vi "camera_grayscale.vi"(0 "Camera configuration":string="{\n     \"type\": \"Camera\",\n     \"listen_port\": 8012,\n     \"location\": {\n       \"x\": 0.0,\n       \"y\": 0.0,\n       \"z\": 250.0\n     },\n     \"rotation\": {\n       \"pitch\": 0.0,\n       \"yaw\": 0.0,\n       \"roll\": 0.0\n     },\n     \"stream_dimensions\": {\n       \"x\": 512.0,\n       \"y\": 512.0\n     },\n    \"dynamic_range\": 1.0,\n   \t\"fov\": 60.0,\n    \"camera_matrix\": [\n         [433.0, 0.0,   256.0],\n         [0.0,   433.0, 256.0],\n         [0.0,   0.0,   1.0]\n     ],\t\n   \t\"min_shutter\": 0.0005,\n   \t\"max_shutter\": 0.0014,\n    \"motion_blur_bias\": 0.1,\n    \"white_balance\": 0.0,\n    \"white_balance_temp_offset\": 0,\n    \"exposure_compensation\": -1.0,\n    \"image_noise_bias\": 0.05,\n    \"ray_tracing\":{\n       \"enable_ray_tracing\": false\n    },\n   \"channels\" : \"gray\",\n   \"annotation\": {\n      \"include_annotation\": false,\n      \"desired_tags\": [\n        \"traffic_sign\", \"vehicle\"\n      ],\n     \"include_lanes\": true,\n\t\t    \"lane_sampling_distance\": 15000.0,\n\t\t    \"lane_sampling_frequency\": 100.0,\n\t\t    \"lane_subsampling\": 10.0,\n      \"far_plane\": 10000.0,\n      \"include_tags\": true,\n      \"include_obb\": false,\n      \"cull_partial_frame\":false,\n      \"debug_draw\":false\n    },\n    \"max_distance\":50000.0,\n    \"channel_depth\":1\n}\n", 3 "error In":errorcluster={"status"=FALSE, "code"=0, "source"="Event Code: 0\r\n\r\n-----------------------------------\nEvent Code: 0\r\n{\"message\":\"Successfully configured scenario.\",\"reference\":973,\"success\":true,\"type\":\"ClosedLoopConfigCommand_ID\"}\r\n-----------------------------------\nEvent Code: 0\r\n{\"message\":\"weather configured to \\\"Default\\\"\",\"reference\":703,\"success\":true,\"type\":\"WeatherConfig\"}\r\n-----------------------------------\nEvent Code: 0\r\n{\"message\":\"complete\",\"reference\":874,\"success\":true,\"type\":\"REPLAY_ConfigureSensorsCommand_ID\"}\r\n-----------------------------------\n"}) -> (4 "Camera configuration":string="{\n     \"type\": \"Camera\",\n     \"listen_port\": 8012,\n     \"location\": {\n       \"x\": 0.0,\n       \"y\": 0.0,\n       \"z\": 250.0\n     },\n     \"rotation\": {\n       \"pitch\": 0.0,\n       \"yaw\": 0.0,\n       \"roll\": 0.0\n     },\n     \"stream_dimensions\": {\n       \"x\": 512.0,\n       \"y\": 512.0\n     },\n    \"dynamic_range\": 1.0,\n   \t\"fov\": 60.0,\n    \"camera_matrix\": [\n         [433.0, 0.0,   256.0],\n         [0.0,   433.0, 256.0],\n         [0.0,   0.0,   1.0]\n     ],\t\n   \t\"min_shutter\": 0.0005,\n   \t\"max_shutter\": 0.0014,\n    \"motion_blur_bias\": 0.1,\n    \"white_balance\": 0.0,\n    \"white_balance_temp_offset\": 0,\n    \"exposure_compensation\": -1.0,\n    \"image_noise_bias\": 0.05,\n    \"ray_tracing\":{\n       \"enable_ray_tracing\": false\n    },\n   \"channels\" : \"gray\",\n   \"annotation\": {\n      \"include_annotation\": false,\n      \"desired_tags\": [\n        \"traffic_sign\", \"vehicle\"\n      ],\n     \"include_lanes\": true,\n\t\t    \"lane_sampling_distance\": 15000.0,\n\t\t    \"lane_sampling_frequency\": 100.0,\n\t\t    \"lane_subsampling\": 10.0,\n      \"far_plane\": 10000.0,\n      \"include_tags\": true,\n      \"include_obb\": false,\n      \"cull_partial_frame\":false,\n      \"debug_draw\":false\n    },\n    \"max_distance\":50000.0,\n    \"channel_depth\":1\n}\n", 6 "Image":picture, 7 "Raw data":u8[](array[numeric]), 8 "Annotation Data":string, 9 "error out":errorcluster={"status"=TRUE, "code"=1, "source"="Error Code: 1\r\nTCP Write in mono_send_command.vi->mono_camera_grayscale.vi\r\n-----------------------------------\nError Code: 0\r\n\r\n-----------------------------------\n"})   [LabVIEW 2019]
doc: "Configures and reads the data stream for a Grayscale Camera sensor and outputs a picture with the specified format in the stream dimensions."
uses:
  tools/simx_common.vi
  controls/Header.ctl
panel:
  out "Header":T1={"length"=262160, "time_stamp"=1617235638, "game_time"=1137806000.0, "frame_count"=367} {"game_time" format="%_10g"}
  in  "Show Annotation":bool
  in  "null connection":refnum<k5>
  in  "camera_connection":refnum<k5>
  # "Note: set annotation settings in camera configuration json"
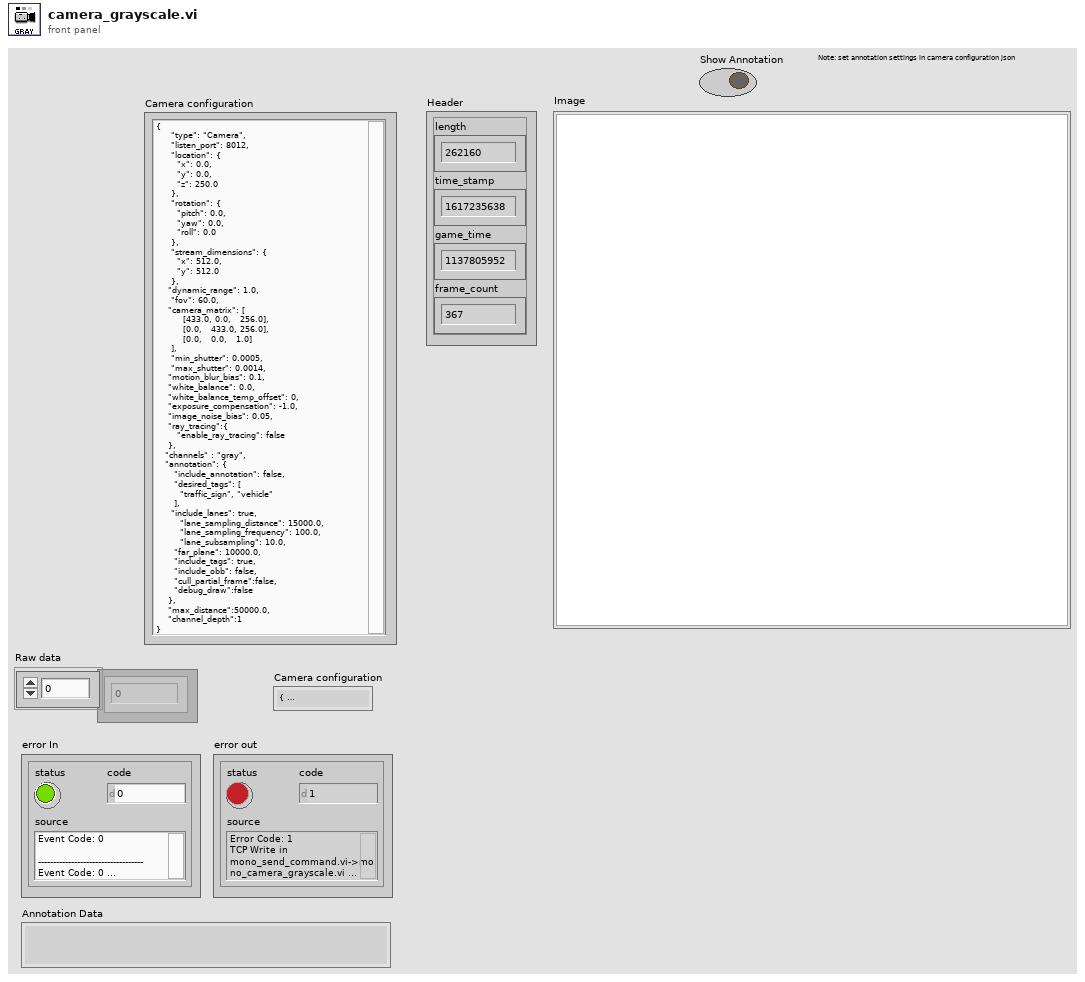
[diagram p1: front panel]
types:
  T1 = typedef "Header.ctl" = cluster{"length":u32, "time_stamp":u32, "game_time":sgl, "frame_count":u32}
  T2 = typedef "simx_connection.ctl" = cluster{"Config":T3, "Connections":T6, "Map":cluster{"lanes":cluster{"x":dbl[], "y":dbl[], "z":dbl[]}, "StartPosition":cluster{"start_points":T7, "StartRotation":dbl[], "StartLocation":dbl[]}, "Draw Map Size":T8, "DrawArea":cluster{"min_Y":dbl, "min_X":dbl, "Scale X":dbl, "Scale Y":dbl}, "Map":picture, "Map Geojson":string}}
  T3 = typedef "config.ctl" = cluster{"Trajectory":T4, "Weather":T5}
  T4 = typedef "trajectory.ctl" = cluster{"Number of frames":i32, "Frame number":i32, "Trajectory":string}
  T5 = typedef "weather.ctl" = cluster{"id":string}
  T6 = typedef "connections.ctl" = cluster{"Simulator Connection":refnum<k5>, "server_ip":string, "Port":i32, "Sensor connections":refnum<k5>[]}
  T7 = typedef "start_points.ctl" = cluster{"locations":dbl[][], "rotations":dbl[][], "type":string[]}
  T8 = typedef "LVBoundsTypeDef.ctl" = cluster{"Width":u32, "Height":u32}
  T9 = typedef "sensor_sample.ctl" = cluster{"Header":T1, "data out":string}
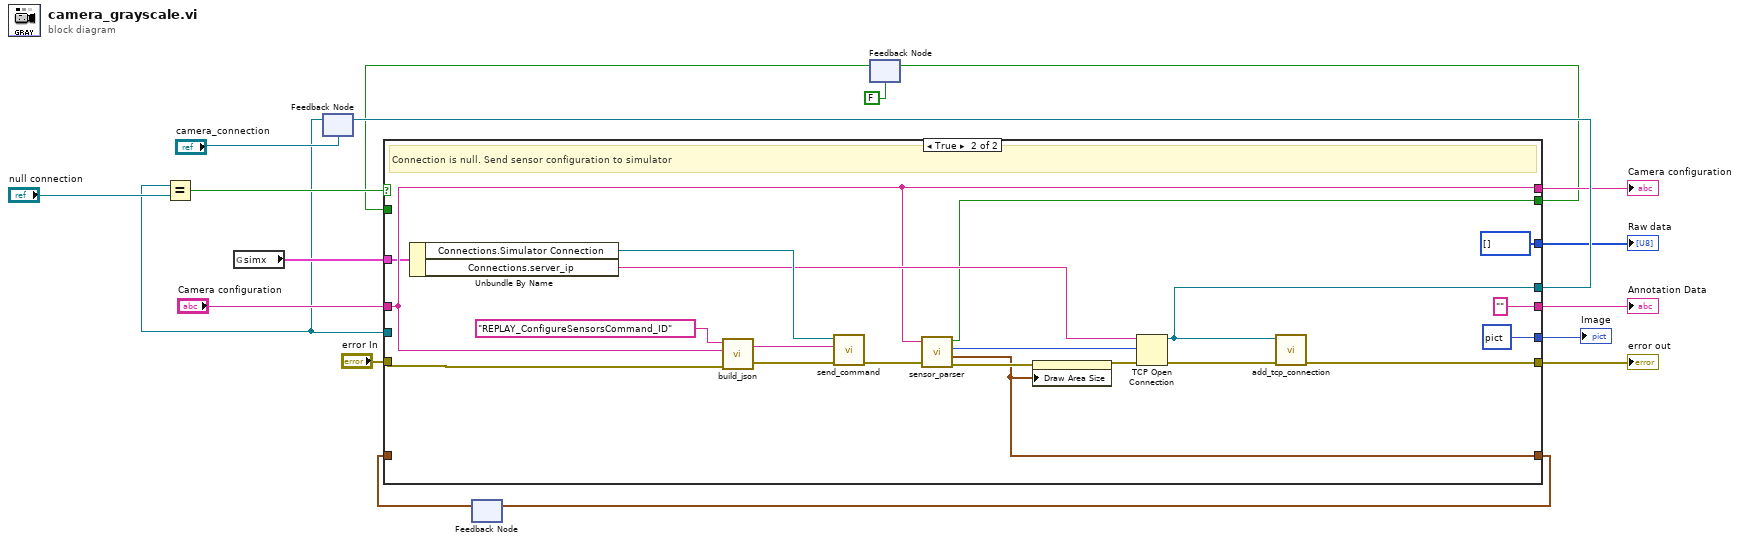
[diagram p0: block diagram]
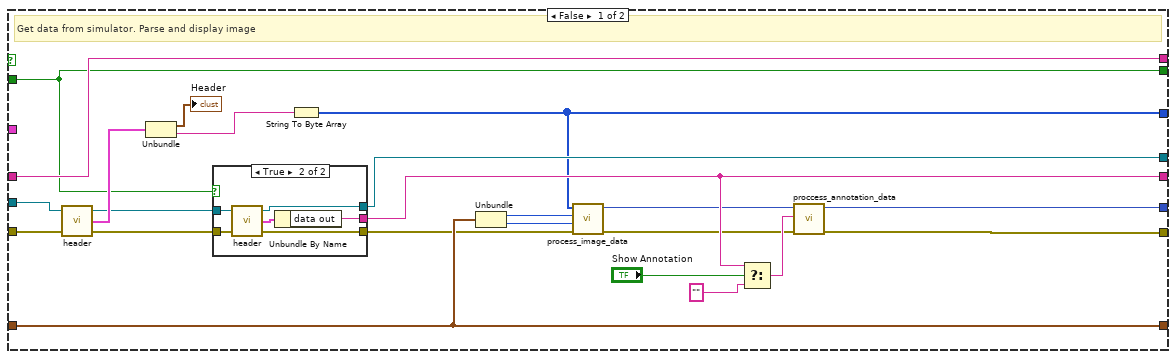
[diagram p2: hidden frame]
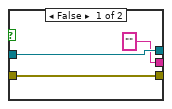
[diagram p3: hidden frame]
diagram:
  n1 = global read "simx_common.vi" "simx"() -> (w2:T2)
  n2 = feedback #1("camera_connection") -> (w1:refnum<k5>)
  n3 = Equal?(x=w1, y="null connection") -> (x = y?=w15:bool)
  n4 = feedback #2() -> (w10:cluster{"x dimension":i32, "y dimension":i32})  [unwired: 1 in]
  n5 = feedback #3(FALSE) -> (w4:bool)
  n6 = case shown="True" w15 {
    tunnel: [w34 w51] -> w13
    tunnel: "Camera configuration" -> [w36 w55]
    tunnel: [w26 w53] -> w16
    tunnel: w1 -> [w39 _]
    tunnel: "error In" -> [w38 w61]
    tunnel: w10 -> [w37 _]
    tunnel: [w33 picture data[5B] ("new picture")] -> w7
    tunnel: [w37 w58] -> w11
    tunnel: [w22 u8[] [] ("unsigned byte array")] -> w9
    tunnel: [w36 w55] -> w8
    tunnel: [w35 w57] -> w6
    tunnel: w4 -> [w35 _]
    tunnel: [w32 "" ("data out")] -> w3
    tunnel: w2 -> [_ w54]
    frame False {
      # "Get data from simulator. Parse and display image"
      n7 = call "header.vi"("error in"=w38, "TCP Network Connection in"=w39) -> ("error out"=w23:errorcluster, "Sensor sample"=w40:T9, "TCP Network Connection out"=w30:refnum<k5>)  [unwired: 1 in]
      n8 = Unbundle(w40) -> ("Header"=→"Header":T1, "data out"=w41:string)
      n9 = case shown="True" w35 {
        tunnel: w30 -> [w44 w50]
        tunnel: [w44 w49] -> w26
        tunnel: w23 -> [w42 w48]
        tunnel: ["" ("data out") w46] -> w32
        tunnel: [w42 w45] -> w25
        frame False {
        }
        frame True {
          n10 = call "header.vi"("error in"=w48, "TCP Network Connection in"=w50) -> ("error out"=w45:errorcluster, "Sensor sample"=w47:T9, "TCP Network Connection out"=w49:refnum<k5>)  [unwired: 1 in]
          n11 = Unbundle By Name(w47) -> ("data out"=w46:string)
        }
      }
      n12 = String To Byte Array(string=w41) -> (unsigned byte array=w22:u8[])
      n13 = Unbundle(w37) -> ("x dimension"=w21:i32, "y dimension"=w20:i32)
      n14 = call "process_image_data.vi"("error in"=w25, "y"=w20, "x"=w21, "Raw data"=w22) -> ("error out"=w24:errorcluster, "Image"=w19:picture)  [unwired: 4 in]
      n15 = Select(t=w32, s="Show Annotation", f="") -> (s? t:f=w27:string)
      n16 = call "proccess_annotation_data.vi"("error in"=w24, "Annotation Data"=w27, "Image in"=w19) -> ("error out"=w34:errorcluster, "Image out"=w33:picture)  [unwired: 2 in, 1 out]
    }
    frame True {
      # "Connection is null. Send sensor configuration to simulator"
      n17 = Unbundle By Name(w54) -> ("Connections.Simulator Connection"=w64:refnum<k5>, "Connections.server_ip"=w62:string)
      n18 = call "build_json.vi"("error in"=w61, "Message"=w55, "Command_ID"="REPLAY_ConfigureSensorsCommand_ID") -> ("error out"=w68:errorcluster, "JSON Out"=w69:string)  [unwired: 1 in]
      n19 = call "send_command.vi"("error in"=w68, "JSON Command"=w69, "TCP Network Connection in"=w64) -> ("error out"=w60:errorcluster)  [unwired: 1 in, 3 out]
      n20 = call "sensor_parser.vi"("Sensor configuration"=w55, "error in"=w60) -> ("include_annotation"=w57:bool, "Port out"=w56:u16, "Stream dimensions"=w58:cluster{"x dimension":i32, "y dimension":i32}, "error out"=w59:errorcluster)  [unwired: 1 in]
      n21 = property on="Image" class="Pict"(error in=w59, "Draw Area Size"=w58) -> (error out=w63:errorcluster)  [unwired: 1 in, 1 out]
      n22 = TCP Open Connection(address=w62, remote port or service name=w56, error in (no error)=w63) -> (connection ID=w53:refnum<k5>, error out=w52:errorcluster)  [unwired: 2 in]
      n23 = call "add_tcp_connection.vi"("error in"=w52, "Sensor connection"=w53) -> ("error out"=w51:errorcluster)  [unwired: 5 in]
    }
  }
  "error out" <- w13
  "Image" <- w7
  "Raw data" <- w9
  "Camera configuration" <- w8
  "Annotation Data" <- w3
  n24 = feedback-in #1(w16) -> ()
  n25 = feedback-in #2(w11) -> ()
  n26 = feedback-in #3(w6) -> ()
